vi "Spartan HTTP Write Session Data.vi"(4 "error in (no error)":errorcluster, 6 "data":string, 7 "http session":T1 {"object data"."time" format="%0.2f"}) -> (0 "error out":errorcluster, 3 "http session out":T1 {"object data"."time" format="%0.2f"})   [LabVIEW 2011]
uses:
  Spartan HTTP Session.ctl
  Addons/internet/http/http_obj.llb/HTTP Session Data.ctl
  Addons/internet/utils/keyedarr.llb/Keyed Array.ctl
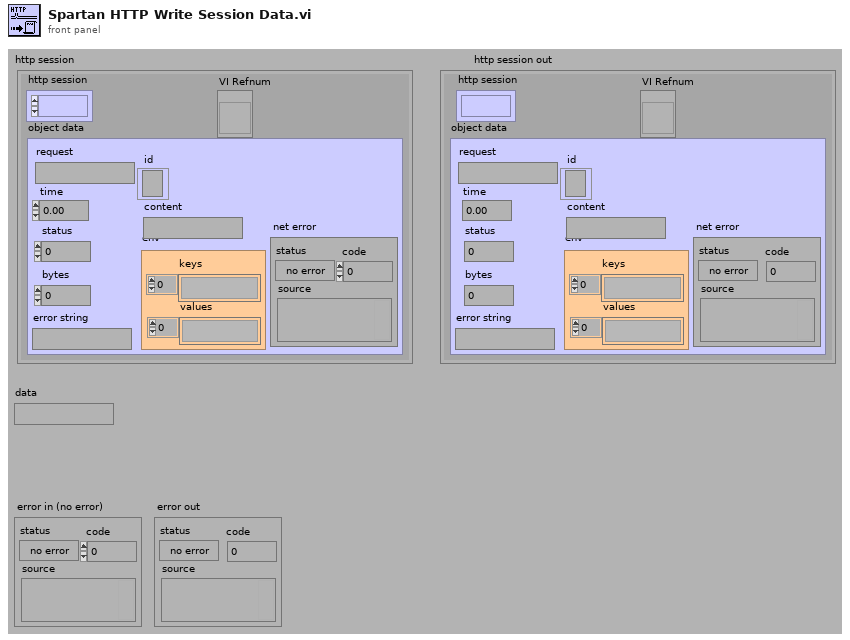
[diagram p1: front panel]
types:
  T1 = typedef "Spartan HTTP Session.ctl" = cluster{"http session":refnum<k1>, "object data":T2, "VI Refnum":refnum<vi>}
  T2 = typedef "HTTP Session Data.ctl" = cluster{"request":string, "time":dbl, "status":i32, "error string":string, "bytes":i32, "env":T3, "content":string, "id":refnum<k5>, "net error":errorcluster}
  T3 = typedef "Keyed Array.ctl" = cluster{"keys":string[], "values":string[]}
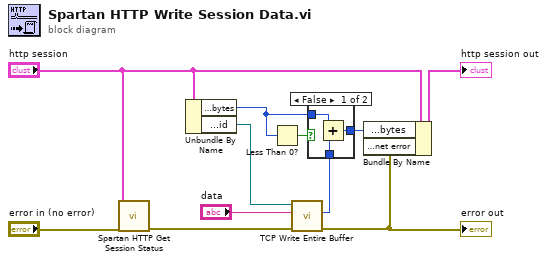
[diagram p0: block diagram]
diagram:
  n1 = call "Spartan HTTP Get Session Status.vi"("error in (no error)"="error in (no error)", "http session"="http session") -> ("error out"=w2:errorcluster)  [unwired: 9 out]
  n2 = Unbundle By Name("http session") -> ("object data.bytes"=w5:i32, "object data.id"=w1:refnum<k5>)
  n3 = Less Than 0?(x=w5) -> (x < 0?=w6:bool)
  n4 = call "TCP Write Entire Buffer.vi"("error in (no error)"=w2, "data in"="data", "connection ID"=w1) -> ("error out"=w10:errorcluster, "bytes written"=w3:i32)  [unwired: 7 out]
  "error out" <- w10
  n5 = case shown="False" w6 {
    tunnel: w5 -> [w14 _]
    tunnel: [w13 w15] -> w4
    tunnel: w3 -> [w12 w15]
    frame False {
      n6 = Add(x=w14, y=w12) -> (x+y=w13:i32)
    }
    frame True {
    }
  }
  n7 = Bundle By Name(cluster="http session", "object data.bytes"=w4, "object data.net error"=w10) -> (→"http session out":T1)
